vi "Loadingscreen_171213.vi"(11 "2D Picture":picture) -> (3 "2D Picture 2":picture)   [LabVIEW 2016]
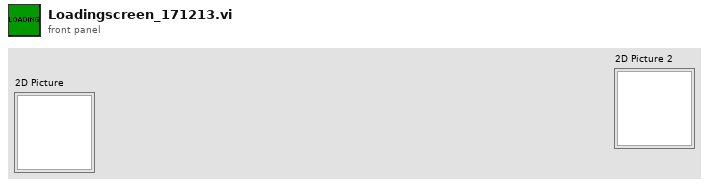
[diagram p1: front panel]
types:
  T1 = cluster{"left":i16, "top":i16, "right":i16, "bottom":i16}
  T2 = cluster{"Font Name:":string, "Size":i16, "Strikeout?":bool, "Italic?":bool, "Underline?":bool, "Outline?":bool, "Shadow?":bool, "Bold?":bool}
  T3 = enum16{"User-specified Font", "Application Font", "System Font", "Dialog Font"}
  T4 = enum16{"None", "Stacked", "Clockwise", "Counterclockwise"}
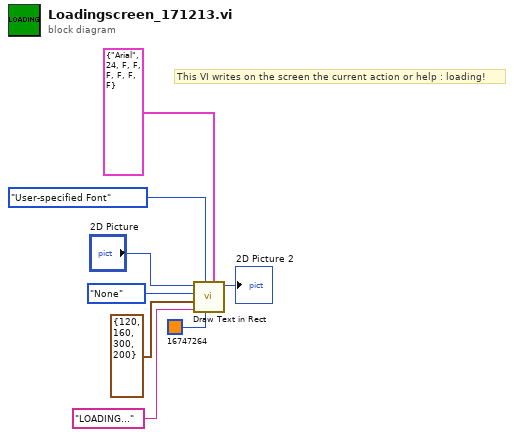
[diagram p0: block diagram]
diagram:
  # "This VI writes on the screen the current action or help : loading!"
  n1 = call <vilib>:"Draw Text in Rect.vi"("[user-specified font]"=T2 {"Font Name:"="Arial", "Size"=24, "Strikeout?"=FALSE, "Italic?"=FALSE, "Underline?"=FALSE, "Outline?"=FALSE, "Shadow?"=FALSE, "Bold?"=FALSE}, "text color(black)"=u32 16747264, "desired font(Application)"=T3."User-specified Font", "text"="LOADING...", "rect"=T1 {"left"=120, "top"=160, "right"=300, "bottom"=200}, "text orientation"=T4."None", "picture"="2D Picture") -> ("new picture"=→"2D Picture 2":picture)  [unwired: 4 in]
